vi "Test Snake Can Eat.vi"(8 "error in (no error)":errorcluster, 11 "Test Case In":refnum<class "Snake Test.lvclass">) -> (0 "error out":errorcluster, 3 "Test Case Out":refnum<class "Snake Test.lvclass">)   [LabVIEW 2020, in "Snake Test.lvclass"]
uses:
  Snake Test.lvclass
  C:/Program Files (x86)/National Instruments/LabVIEW 2020/vi.lib/Astemes/LUnit/Test Case.lvclass
  source/Snake/Direction.ctl
  source/Particle/Position.ctl
  <vilib>/Astemes/LUnit/Test Case.lvclass/Test Case.ctl
  <vilib>/Astemes/LUnit/Palette/Fail.vi
  <vilib>/Astemes/LUnit/Palette/Pass.vi
  <vilib>/Astemes/LUnit/Set Assertion Type.vi
  <vilib>/Astemes/LUnit/Add test result.vi
  <vilib>/Astemes/LUnit/LUnit Record Assertion Result.vi
  <vilib>/Astemes/LUnit/LUnit Aggregate Assertion Results.vi
  <vilib>/Astemes/LUnit/Method Result/LUnit Merge Status.vi
  <vilib>/Astemes/LUnit/LUnit Concatenate result strings.vi
  Snake Test.lvclass/Snake Test.ctl
  source/Snake/Snake.lvclass
  source/Particle.lvclass
  <vilib>/Astemes/LUnit/Test Case.lvclass
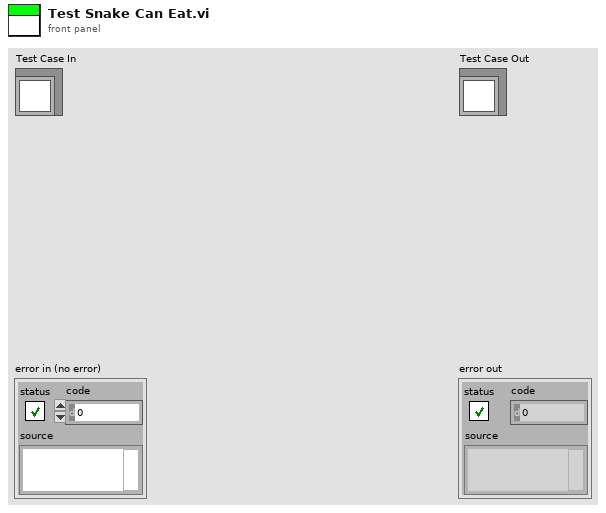
[diagram p1: front panel]
types:
  T1 = typedef "Particle.lvclass/Position.ctl" = cluster{"X":i32, "Y":i32}
  T2 = typedef "Direction.ctl" = enum16{"X", "-X", "Y", "-Y"}
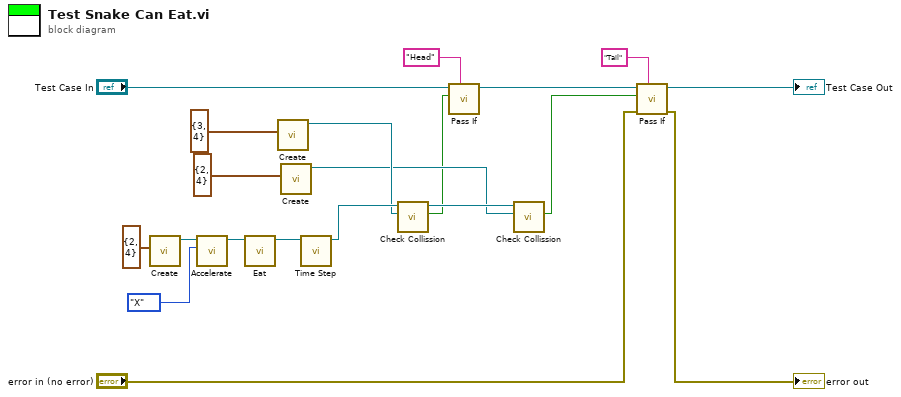
[diagram p0: block diagram]
diagram:
  n1 = call "Create.vi"("Position"=T1 {"X"=2, "Y"=4}) -> ("Snake out"=w16:refnum<class "Snake.lvclass">)  [unwired: 10 in]
  n2 = call "Accelerate.vi"("Direction"=Direction."X", "Snake in"=w16) -> ("Snake out"=w13:refnum<class "Snake.lvclass">)  [unwired: 9 in]
  n3 = call "Eat.vi"("Snake in"=w13) -> ("Snake out"=w14:refnum<class "Snake.lvclass">)  [unwired: 9 in, 1 out]
  n4 = call "Create.vi"("Position"=T1 {"X"=3, "Y"=4}) -> ("Particle out"=w8:refnum<class "Particle.lvclass">)  [unwired: 10 in]
  n5 = call "Create.vi"("Position"=T1 {"X"=2, "Y"=4}) -> ("Particle out"=w6:refnum<class "Particle.lvclass">)  [unwired: 10 in]
  n6 = call "Time Step.vi"("Snake in"=w14) -> ("Snake out"=w11:refnum<class "Snake.lvclass">)  [unwired: 10 in]
  n7 = call "Check Collission.vi"("Particle"=w8, "Snake in"=w11) -> ("Collided?"=w4:bool, "Snake out"=w10:refnum<class "Snake.lvclass">)  [unwired: 8 in]
  n8 = call <vilib>:"Pass If.vi"("Description"="Head", "Pass?"=w4, "LUnit Test Case In"="Test Case In") -> ("LUnit Test Case Out"=w5:refnum<class "Snake Test.lvclass">)  [unwired: 7 in, 1 out]
  n9 = call "Check Collission.vi"("Particle"=w6, "Snake in"=w10) -> ("Collided?"=w3:bool)  [unwired: 8 in, 1 out]
  n10 = call <vilib>:"Pass If.vi"("Description"="Tail", "error in (no error)"="error in (no error)", "Pass?"=w3, "LUnit Test Case In"=w5) -> ("error out"=→"error out":errorcluster, "LUnit Test Case Out"=→"Test Case Out":refnum<class "Snake Test.lvclass">)  [unwired: 6 in]
